vi "Get Bmp Info Header.vi"(8 "错误输入":errorcluster, 9 "偏移量(0)":i32, 11 "Bmp Data In":string) -> (0 "错误输出":errorcluster, 1 "Offset":i32, 2 "Info Header":T1, 3 "Bmp Data Out":string)   [LabVIEW 2012, in "Picture Box Tools.lvlib" / "BMP File.lvlib"]
uses:
  BMP File.lvlib
  Bmp Info Header.ctl
panel:
  in  "Bitmap-Info Header":T1
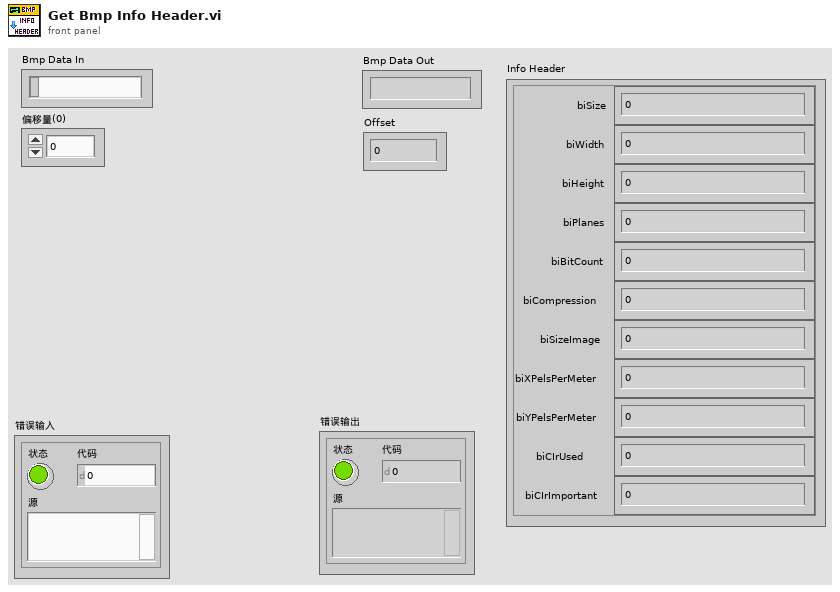
[diagram p1: front panel]
types:
  T1 = typedef "Picture Box Tools.lvlib/BMP File.lvlib/Bmp Info Header.ctl" = cluster{"biSize":u32, "biWidth":i32, "biHeight":i32, "biPlanes":u16, "biBitCount":u16, "biCompression":u32, "biSizeImage":u32, "biXPelsPerMeter":i32, "biYPelsPerMeter":i32, "biCIrUsed":u32, "biCIrImportant":u32}
  T2 = enum16{"big-endian, network order", "native, host order", "little-endian"}
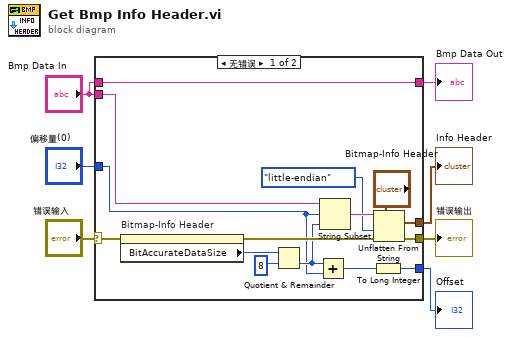
[diagram p0: block diagram]
diagram:
  n1 = case shown="无错误" "错误输入" {
    selector: "错误输入" -> [w21 w23]
    tunnel: "偏移量(0)" -> [w9 _]
    tunnel: "Bmp Data In" -> [w22 _]
    tunnel: [w18 _] -> w1
    tunnel: [w16 w23] -> w6
    tunnel: "Bmp Data In" -> [w15 w24]
    tunnel: [w15 w24] -> w4
    tunnel: [w10 _] -> w2
    frame No Error {
      n2 = property on="Bitmap-Info Header" class="Clust (严格)"(error in=w21) -> (error out=w17:errorcluster, "BitAccurateDataSize"=w13:u32)  [unwired: 1 in, 1 out]
      n3 = Quotient & Remainder(x=w13, y=u32 8) -> (floor(x/y)=w11:u32)  [unwired: 1 out]
      n4 = Add(x=w11, y=w9) -> (x+y=w14:u32)
      n5 = String Subset(string=w22, offset (0)=w9, length (rest)=w11) -> (substring=w20:string)
      n6 = To Long Integer(number=w14) -> (32bit integer=w10:i32)
      n7 = Unflatten From String(type="Bitmap-Info Header", binary string=w20, byte order (0:big-endian, network order)=T2."little-endian" ("字节顺序(0:big-endian, network order)"), error in (no error)=w17) -> (value=w18:T1, error out=w16:errorcluster)  [unwired: 1 in, 1 out]
    }
    frame Error {
    }
  }
  "错误输出" <- w6
  "Bmp Data Out" <- w4
  "Offset" <- w2
  "Info Header" <- w1
